vi "MathCAD variables.vi"(8 "error in (no error)":errorcluster, 10 "MathCAD variables":T1) -> (0 "error out":errorcluster, 2 "MathCAD results":T2)   [LabVIEW 2015]
uses:
  <vilib>/Utility/file.llb/Read From Spreadsheet File (string).vi
  <vilib>/Utility/config.llb/NI_LVConfig.lvlib
  <vilib>/Utility/config.llb/Read Key (Boolean).vi
  Variable cluster.ctl
  MathCAD results ref.ctl
panel:
  in  "MathCAD results constant":T2
  out "languages":i32
  out "all rows":string[][](array[string])
  out "first row":string[](array[string])
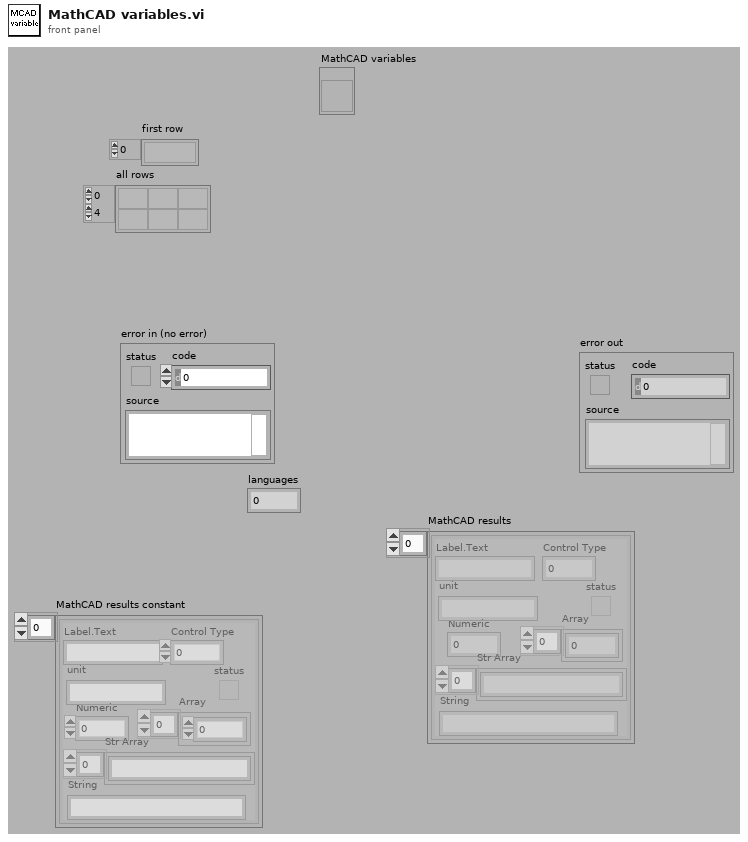
[diagram p1: front panel]
types:
  T1 = typedef "MathCAD results ref.ctl" = refnum<vi>
  T2 = typedef "Variable cluster.ctl" = cluster{"Label.Text":string, "Control Type":u32, "Numeric":dbl, "Array":dbl[], "status":bool, "Str Array":string[], "String":string, "unit":string}[]
  T3 = typedef "NI_LVConfig.lvlib/Config Data RefNum.ctl" = refnum<k1>
  T4 = cluster{"Label.Text":string, "Control Type":u32, "Numeric":dbl, "Array":dbl[], "status":bool, "Str Array":string[], "String":string, "unit":string}
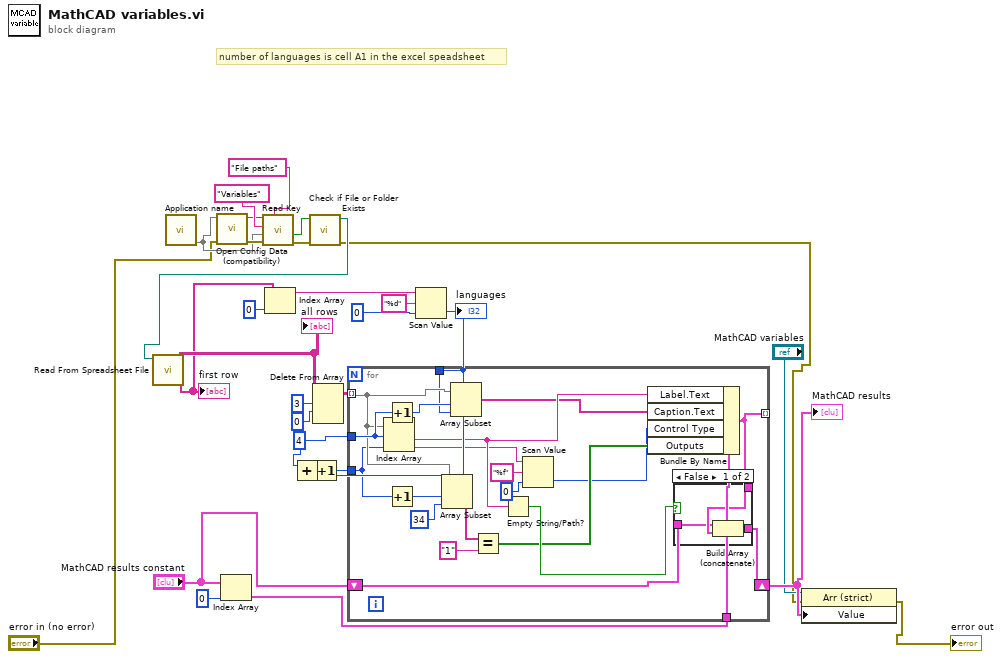
[diagram p0: block diagram]
diagram:
  w18 = 4 ("index")
  # "number of languages is cell A1 in the excel speadsheet"
  n1 = call "Application name.vi"() -> (0:w5)  [unwired: 4 in, 3 out]
  n2 = call <vilib>:"Open Config Data (compatibility).vi"("error in (no error)"="error in (no error)", "configuration file path"=w5) -> ("error out"=w8:errorcluster, "refnum"=w4:T3)  [unwired: 7 in, 1 out]
  n3 = Index Array(array="MathCAD results constant", index=0) -> (element=w13:T4)
  n4 = call-poly <vilib>:"Read Key.vi"("section"="File paths", "error in (no error)"=w8, "default value"=w5, "key"="Variables", "refnum"=w4) -> ("error out"=w7:errorcluster, "value"=w9:bool)  [unwired: 3 in, 2 out]
  n5 = call <vilib>:"Check if File or Folder Exists.vi"("error in (no error)"=w7, "path"=w9) -> ("error out"=w2:errorcluster, "dup path"=w3:path)  [unwired: 7 in, 1 out]
  n6 = call-poly <vilib>:"Read From Spreadsheet File.vi"("file path (dialog if empty)"=w3) -> ("first row"=w23:string[], "all rows"=w28:string[][])  [unwired: 6 in, 3 out]
  "first row" <- w23
  "all rows" <- w28
  n7 = Index Array(array=w23, index=0) -> (element=w21:string)
  n8 = Delete From Array(array=w28, length=3, index (row)=0) -> (array with subset deleted=w25:string[][])  [unwired: 1 in, 1 out]
  n9 = Scan Value(string=w21, format string="%d", default (0 dbl)=0) -> (value=w17:i32)  [unwired: 1 out]
  "languages" <- w17
  n10 = Add(x=w18, y=w17) -> (x+y=w19:i32)
  n11 = Increment(x=w19) -> (x+1=w16:i32)
  n12 = for {
    tunnel: w25 -> [w39] mode=indexing
    tunnel: [w46] -> _ mode=indexing
    shift-right: [w50] -> w12
    shift-left: "MathCAD results constant" -> [w41]
    tunnel: w18 -> [w43]
    tunnel: w16 -> [w33]
    tunnel: w17 -> [w34]
    tunnel: w13 -> [w40]
    n13 = Index Array(array=w39, index #1=w43, index #2=w33) -> (element #1=w48:string, element #2=w45:string)
    n14 = Increment(x=w43) -> (x+1=w42:i32)
    n15 = Increment(x=w33) -> (x+1=w32:i32)
    n16 = Array Subset(array=w39, index=w32, length=34) -> (w37:string[])
    n17 = Array Subset(array=w39, index=w42, length=w34) -> (w44:string[])
    n18 = Equal?(x=w37, y="1") -> (x = y?=w35:bool[])
    n19 = Empty String/Path?(string/path=w48) -> (empty?=w47:bool)
    n20 = Scan Value(string=w45, format string="%f", default (0 dbl)=u32 0 ("Control Type")) -> (value=w31:u32)  [unwired: 1 out]
    n21 = Bundle By Name(cluster=w40, "Label.Text"=w48, "Caption.Text"=w44, "Control Type"=w31, "Outputs"=w35) -> (w46:T4)
    n22 = case shown="False" w47 {
      tunnel: w46 -> [w53 _]
      tunnel: w41 -> [w52 w54]
      tunnel: [w51 w54] -> w50
      frame False {
        n23 = Build Array (concatenate)(w52, w53) -> (w51:T2)
      }
      frame True {
      }
    }
  }
  "MathCAD results" <- w12
  n24 = property class="Arr (strict)"(reference="MathCAD variables", error in=w2, "Value"=w12) -> (error out=→"error out":errorcluster)  [unwired: 1 out]
